vi "main.vi"() -> ()   [LabVIEW 2013]
uses:
  qwtb_lvlib/TD Quantity.ctl
  qwtb_lvlib/TD Calculation Settings.ctl
  qwtb_lvlib/TD Uncertainty Calculation Method.ctl
  qwtb_lvlib/TD Correlation Calculation Settings.ctl
  qwtb_lvlib/TD DOF Calculation Settings.ctl
  qwtb_lvlib/TD MCM Calculation Settings.ctl
  qwtb_lvlib/TD MCM Calculation Method.ctl
  qwtb_lvlib/TD GUI Settings.ctl
  qwtb_lvlib/TD Backend Engine.ctl
  qwtb_lvlib/TD Algorithm Information.ctl
  globals.vi
  <vilib>/Utility/xml.llb/Read From XML File(string).vi
  <vilib>/Utility/xml.llb/Write to XML File(string).vi
panel:
  in  "calculate":bool
  in  "help":bool
  out "error out":errorcluster
  in  "quit":bool
  # "simple QWTB GUI"
  # "see EMRP project Q-Wave"
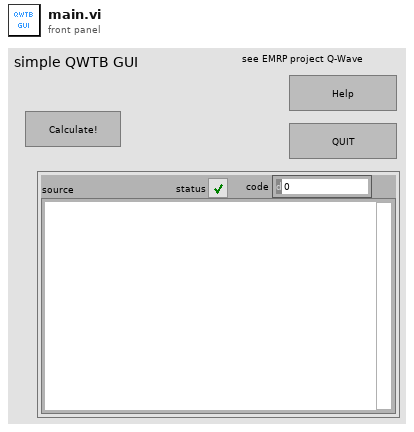
[diagram p1: front panel]
types:
  T1 = typedef "TD Algorithm Information.ctl" = cluster{"ID":string, "Name":string, "Description":string, "Citation":string, "Remarks":string, "License":string, "Requires":string[], "Requires - description":string[], "Returns":string[], "Returns - description":string[], "Provides GUF":bool, "Provides MCM":bool, "Full path":string}
  T2 = typedef "TD GUI Settings.ctl" = cluster{"Backend engine":T3, "QWTB Folder Path":path}
  T3 = typedef "TD Backend Engine.ctl" = enum16{"Matlab by Script node", "GNU Octave by GOLPI"}
  T4 = typedef "TD Calculation Settings.ctl" = cluster{"Verbose":bool, "Uncertainty Calculation Method":T5, "Correlations":T6, "Degrees of Freedom":T7, "MCM Calculation Settings":T8}
  T5 = typedef "TD Uncertainty Calculation Method.ctl" = enum16{"none", "GUF", "MCM"}
  T6 = typedef "TD Correlation Calculation Settings.ctl" = cluster{"Required":bool, "Generate":bool}
  T7 = typedef "TD DOF Calculation Settings.ctl" = cluster{"Required":bool, "Generate":bool}
  T8 = typedef "TD MCM Calculation Settings.ctl" = cluster{"Repeats":i32, "Verbose":bool, "Parallelization method":T9, "Processors":i32, "Temporary directory":string, "Randomize":bool}
  T9 = typedef "TD MCM Calculation Method.ctl" = enum16{"Single Core", "Multi Core", "Multi Station"}
  T10 = typedef "TD Quantity.ctl" = cluster{"Name":string, "Value":dbl[][], "Uncertainty":dbl[][], "Degrees of\nFreedom":dbl[][], "Correlation":dbl[][], "Randomized uncertainty":dbl[][]}
  T11 = cluster{"Calculation Settings":T4, "GUI Settings":T2, "Data In":T10[], "Available Algorithms":T1[], "Current Algorithm":T1, "Data Out":T10[]}
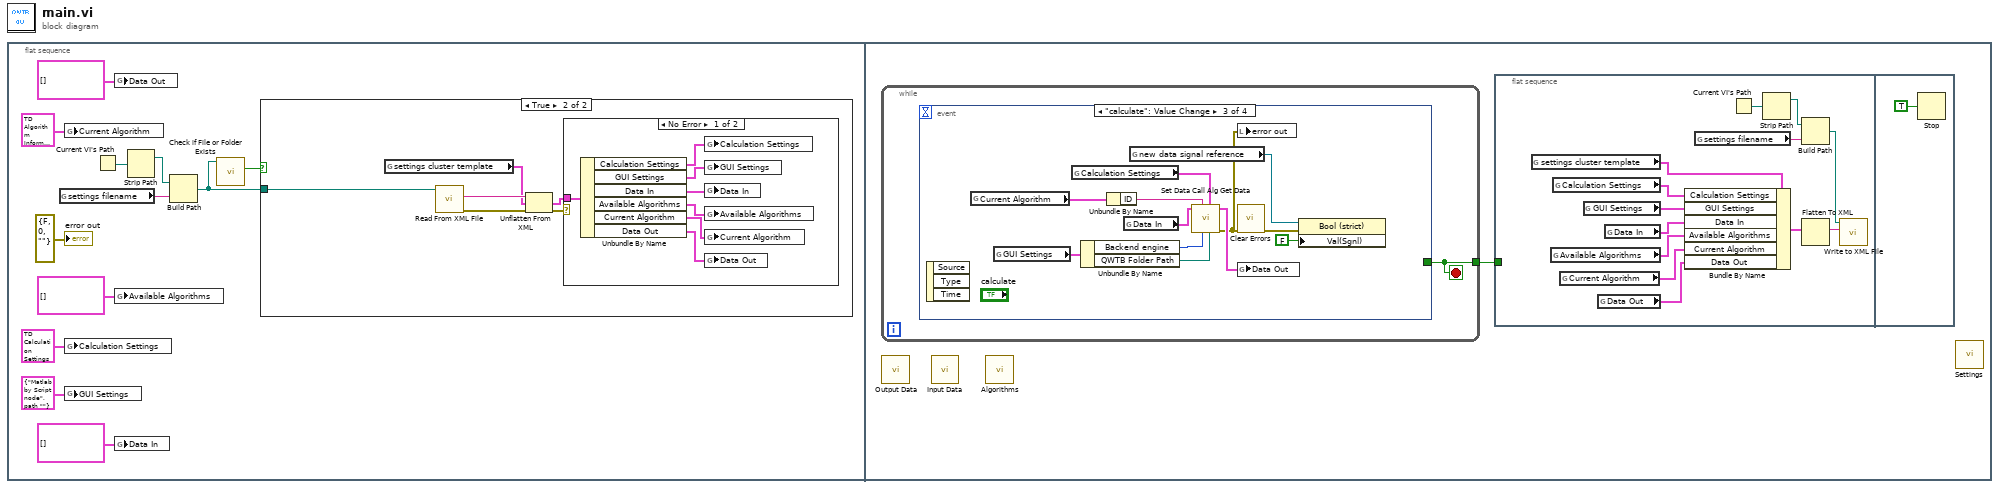
[diagram p0: block diagram]
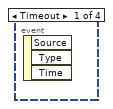
[diagram p4: hidden frame]
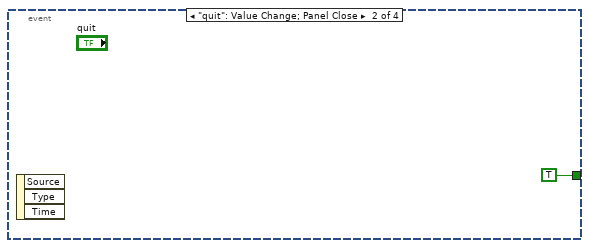
[diagram p5: hidden frame]
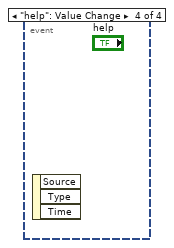
[diagram p6: hidden frame]
diagram:
  n1 = flat-sequence {
    frame #0 {
      n2 = global read "globals.vi" "settings filename"() -> (w5:string)
      n3 = global write "globals.vi" "Current Algorithm"(T1 {"ID"="", "Name"="", "Description"="", "Citation"="", "Remarks"="", "License"="", "Requires"=[], "Requires - description"=[], "Returns"=[], "Returns - description"=[], "Provides GUF"=FALSE, "Provides MCM"=FALSE, "Full path"=""} ("Current Algorithm")) -> ()
      n4 = global write "globals.vi" "Calculation Settings"(T4 {"Verbose"=TRUE, "Uncertainty Calculation Method"=enum."none", "Correlations"={"Required"=FALSE, "Generate"=TRUE}, "Degrees of Freedom"={"Required"=TRUE, "Generate"=TRUE}, "MCM Calculation Settings"={"Repeats"=100, "Verbose"=TRUE, "Parallelization method"=enum."Single Core", "Processors"=1, "Temporary directory"=".", "Randomize"=TRUE}} ("Calculation Settings")) -> ()
      n5 = global write "globals.vi" "GUI Settings"(T2 {"Backend engine"=enum."Matlab by Script node", "QWTB Folder Path"=path ""} ("GUI Settings")) -> ()
      n6 = Current VI's Path() -> (path=w2:path)
      n7 = global write "globals.vi" "Data Out"(T10[] [] ("Data Out")) -> ()
      n8 = global write "globals.vi" "Available Algorithms"(T1[] [] ("Available Algorithms")) -> ()
      n9 = global write "globals.vi" "Data In"(T10[] [] ("Data In")) -> ()
      n10 = Strip Path(path=w2) -> (stripped path=w1:path)  [unwired: 1 out]
      n11 = Build Path(base path=w1, name or relative path=w5) -> (appended path=w3:path)
      n12 = call <vilib>:"Check if File or Folder Exists.vi"("path"=w3) -> ("file or folder exists?"=w4:bool)  [unwired: 8 in, 2 out]
      n13 = case shown="True" w4 {
        tunnel: w3 -> [_ w14]
        frame False {
        }
        frame True {
          n14 = global read "globals.vi" "settings cluster template"() -> (w13:T11)
          n15 = call-poly <vilib>:"Read From XML File.vi"("XML File Path"=w14) -> ("error out"=w17:errorcluster, "XML Elements"=w18:string)  [unwired: 8 in, 1 out]
          n16 = Unflatten From XML(xml string=w18, type=w13, error in (no error)=w17) -> (value=w15:T11, error out=w16:errorcluster)
          n17 = case shown="No Error" w16 {
            tunnel: w15 -> [w25 _]
            frame No Error {
              n18 = Unbundle By Name(w25) -> ("Calculation Settings"=w24:T4, "GUI Settings"=w23:T2, "Data In"=w22:T10[], "Available Algorithms"=w21:T1[], "Current Algorithm"=w20:T1, "Data Out"=w19:T10[])
              n19 = global write "globals.vi" "Calculation Settings"(w24) -> ()
              n20 = global write "globals.vi" "GUI Settings"(w23) -> ()
              n21 = global write "globals.vi" "Data In"(w22) -> ()
              n22 = global write "globals.vi" "Available Algorithms"(w21) -> ()
              n23 = global write "globals.vi" "Current Algorithm"(w20) -> ()
              n24 = global write "globals.vi" "Data Out"(w19) -> ()
            }
            frame Error {
            }
          }
        }
      }
      "error out" <- errorcluster {"status"=FALSE, "code"=0, "source"=""} ("error constant")
    }
    frame #1 {
      n25 = while {
        tunnel: [w41] -> w26
        stop <- w41 stop-if-true
        n26 = event shown="[2] \"calculate\": Value Change" {
          selector: _ -> [_ _ _ _]
          dyn-events: _ -> [_ _ _ _]
          timeout: _ -> [_ _ _ _]
          tunnel: [_ TRUE _ _] -> w41
          event Timeout {
            n27 = event-data() -> ()  [unwired: 1 in, 3 out]
          }
          event "quit": Value Change; Panel Close {
            n28 = event-data() -> ()  [unwired: 1 in, 3 out]
          }
          event "calculate": Value Change {
            n29 = event-data() -> ()  [unwired: 1 in, 3 out]
            n30 = global read "globals.vi" "Current Algorithm"() -> (w44:T1)
            n31 = global read "globals.vi" "GUI Settings"() -> (w49:T2)
            n32 = global read "globals.vi" "Calculation Settings"() -> (w50:T4)
            n33 = Unbundle By Name(w49) -> ("Backend engine"=w48:T3, "QWTB Folder Path"=w47:path)
            n34 = Unbundle By Name(w44) -> ("ID"=w43:string)
            n35 = global read "globals.vi" "Data In"() -> (w54:T10[])
            n36 = global read "globals.vi" "new data signal reference"() -> (w52:refnum<vi>)
            n37 = call "Set Data Call Alg Get Data.vi"("QWTB Folder Path"=w47, "Calculation Settings"=w50, "Backend engine"=w48, "Algorithm ID"=w43, "Data In"=w54) -> ("error out"=w46:errorcluster, "Data Out"=w53:T10[])  [unwired: 5 in]
            n38 = local write "error out"(w46) -> ()
            n39 = call <vilib>:"Clear Errors.vi"("error in (no error)"=w46) -> ("error out"=w45:errorcluster)  [unwired: 6 in]
            n40 = global write "globals.vi" "Data Out"(w53) -> ()
            n41 = property class="Bool (strict)"(reference=w52, error in=w45, "Val(Sgnl)"=FALSE ("Value (Signaling)")) -> ()  [unwired: 2 out]
          }
          event "help": Value Change {
            n42 = event-data() -> ()  [unwired: 1 in, 3 out]
          }
        }
      }
      n43 = call "Output Data.vi"() -> ()  [unwired: 12 in]
      n44 = call "Input Data.vi"() -> ()  [unwired: 12 in]
      n45 = call "Algorithms.vi"() -> ()  [unwired: 12 in]
      n46 = flat-sequence {
        tunnel: w26 -> [_]
        frame #0 {
          n47 = global read "globals.vi" "settings cluster template"() -> (w32:T11)
          n48 = global read "globals.vi" "Available Algorithms"() -> (w36:T1[])
          n49 = global read "globals.vi" "Calculation Settings"() -> (w39:T4)
          n50 = global read "globals.vi" "Current Algorithm"() -> (w35:T1)
          n51 = global read "globals.vi" "GUI Settings"() -> (w38:T2)
          n52 = global read "globals.vi" "Data Out"() -> (w34:T10[])
          n53 = global read "globals.vi" "Data In"() -> (w37:T10[])
          n54 = Bundle By Name(cluster=w32, "Calculation Settings"=w39, "GUI Settings"=w38, "Data In"=w37, "Available Algorithms"=w36, "Current Algorithm"=w35, "Data Out"=w34) -> (w33:T11)
          n55 = global read "globals.vi" "settings filename"() -> (w30:string)
          n56 = Current VI's Path() -> (path=w28:path)
          n57 = Strip Path(path=w28) -> (stripped path=w27:path)  [unwired: 1 out]
          n58 = Build Path(base path=w27, name or relative path=w30) -> (appended path=w31:path)
          n59 = Flatten To XML(anything=w33) -> (xml string=w29:string)
          n60 = call-poly <vilib>:"Write to XML File.vi"("XML Input"=w29, "XML File Path"=w31) -> ()  [unwired: 7 in, 3 out]
        }
        frame #1 {
          n61 = Stop(stop? (T)=TRUE) -> ()
        }
      }
      n62 = call "Settings.vi"() -> ()  [unwired: 12 in]
    }
  }
